vi "ilcbtView.vi"   [LabVIEW 2013, in "ILCBTViews.lvlib"]
uses:
  ILCBTViews.lvlib
  CommandFactory/CommandFactory.lvclass
  UserEvents/UserEvents.lvclass
  UserEvents/UserEvents.lvclass/UserEvents.ctl
  Typedefs/CommandSelector.ctl
  Typedefs/StateSelector.ctl
  Typedefs/ILCBTTypedefs.lvlib
  Controller/Controller.lvclass
  ConfigurationThisComponent/ConfigurationThisComponent.lvclass
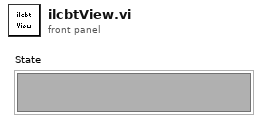
[diagram p1: front panel]
types:
  T1 = enum32{"invalid app kind", "Development System", "Run Time System", "Student Edition", "Embedded LabVIEW", "Evaluation", "Custom"}
  T2 = typedef "ILCBTTypedefs.lvlib/PubDataEvents.ctl" = cluster{"State":refnum<user-event>, "ErrorCode":refnum<user-event>, "OutputData":refnum<user-event>, "LogPath":refnum<user-event>}
  T3 = typedef "ILCBTTypedefs.lvlib/SubDataEvents.ctl" = cluster{"Command":refnum<user-event>}
  T4 = cluster{"Event Registration Refnum":refnum<event-registration>, "Event Registration Refnum":refnum<event-registration>}
  T5 = typedef "ILCBTTypedefs.lvlib/CommandSelector.ctl" = enum16{"ClearError", "Exit", "StandBy", "Start", "Update"}
  T6 = typedef "ILCBTTypedefs.lvlib/StateSelector.ctl" = enum16{"EnabledState", "FaultState", "OffState", "StandbyState"}
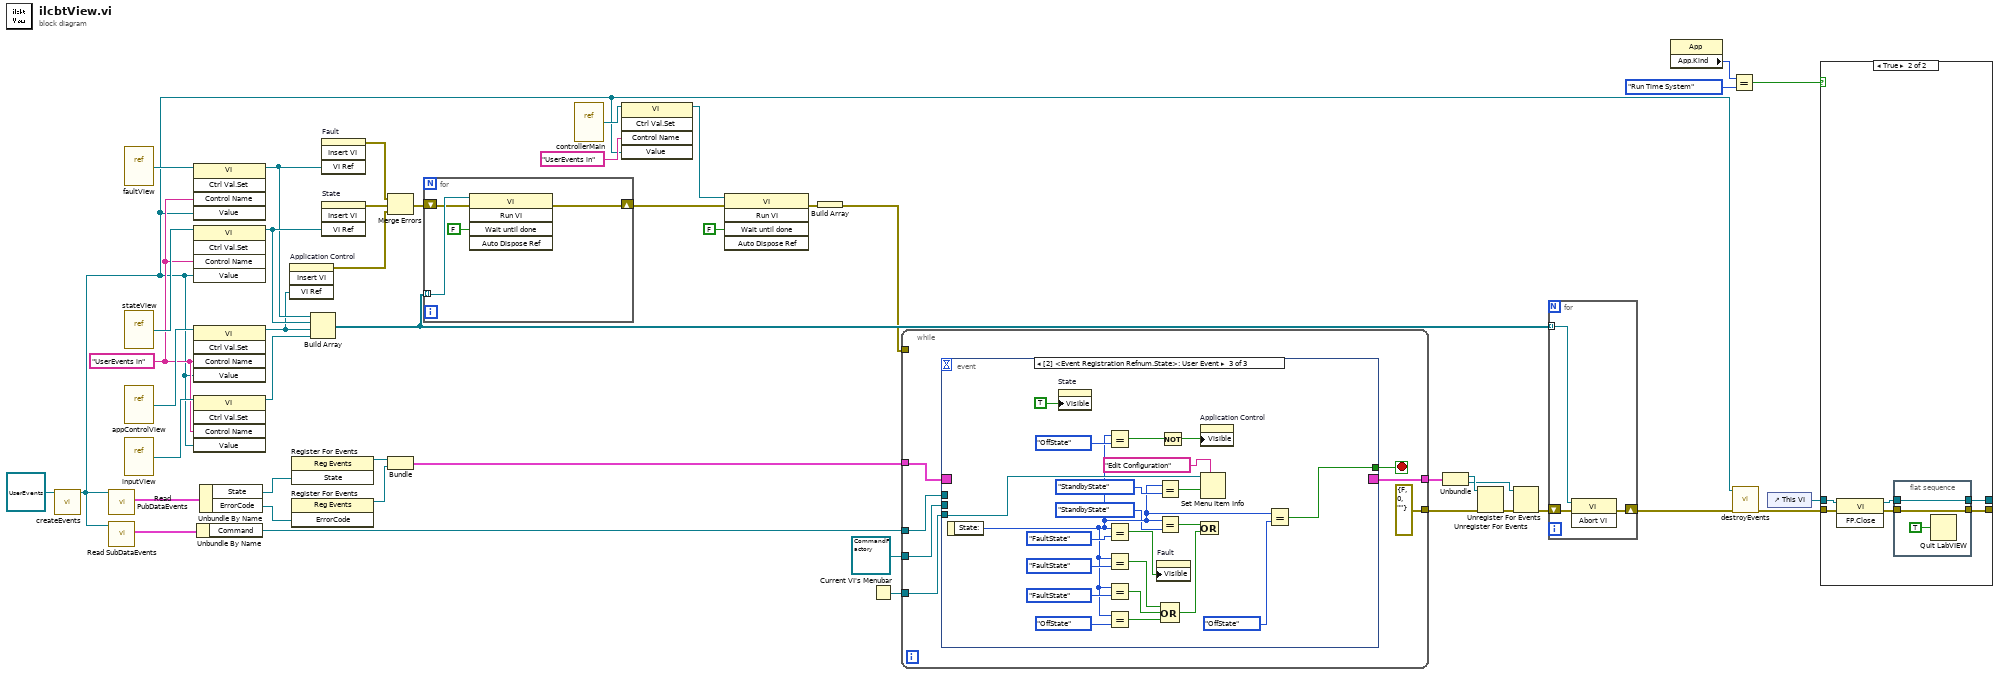
[diagram p0: block diagram]
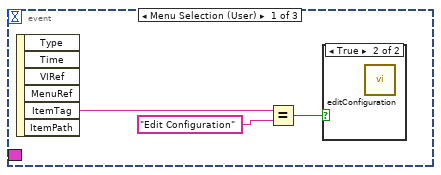
[diagram p3: hidden frame]
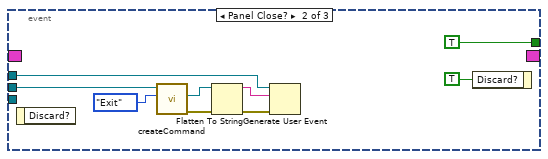
[diagram p5: hidden frame]
diagram:
  w8 = "UserEvents in" ("Control Name")
  n1 = call "createEvents.vi"("UserEvents in"=refnum<class "UserEvents.lvclass"> refnum) -> ("UserEvents out"=w7:refnum<class "UserEvents.lvclass">)  [unwired: 9 in, 1 out]
  n2 = call "Read PubDataEvents.vi"("UserEvents in"=w7) -> ("PubDataEvents"=w38:T2)  [unwired: 9 in, 1 out]
  n3 = call "Read SubDataEvents.vi"("UserEvents in"=w7) -> ("SubDataEvents"=w36:T3)  [unwired: 9 in, 1 out]
  n4 = vi-ref "faultView.vi"() -> (w9:refnum<vi>)
  n5 = vi-ref "stateView.vi"() -> (w12:refnum<vi>)
  n6 = vi-ref "appControlView.vi"() -> (w14:refnum<vi>)
  n7 = vi-ref "inputView.vi"() -> (w26:refnum<vi>)
  n8 = invoke class="VI" method="Ctrl Val.Set"(reference=w9, "Control Name"=w8, "Value"=w7) -> (reference out=w6:refnum<vi>)  [unwired: 2 in, 4 out]
  n9 = invoke class="VI" method="Ctrl Val.Set"(reference=w12, "Control Name"=w8, "Value"=w7) -> (reference out=w11:refnum<vi>)  [unwired: 2 in, 4 out]
  n10 = invoke class="VI" method="Ctrl Val.Set"(reference=w14, "Control Name"=w8, "Value"=w7) -> (reference out=w2:refnum<vi>)  [unwired: 2 in, 4 out]
  n11 = invoke class="VI" method="Ctrl Val.Set"(reference=w26, "Control Name"=w8, "Value"=w7) -> (reference out=w18:refnum<vi>)  [unwired: 2 in, 4 out]
  n12 = Unbundle By Name(w36) -> ("Command"=w35:refnum<user-event>)
  n13 = Unbundle By Name(w38) -> ("State"=w34:refnum<user-event>, "ErrorCode"=w32:refnum<user-event>)
  n14 = invoke on="Application Control" class="SubPnl" method="Insert VI"("VI Ref"=w2) -> (error out=w1:errorcluster)  [unwired: 3 in, 3 out]
  n15 = register-events(w34) -> (reference out=w33:refnum<event-registration>)  [unwired: 2 in, 1 out]
  n16 = register-events(w32) -> (reference out=w31:refnum<event-registration>)  [unwired: 2 in, 1 out]
  n17 = Build Array(w6, w11, w2, w18) -> (w41:refnum<vi>[])
  n18 = invoke on="Fault" class="SubPnl" method="Insert VI"("VI Ref"=w6) -> (error out=w5:errorcluster)  [unwired: 3 in, 3 out]
  n19 = invoke on="State" class="SubPnl" method="Insert VI"("VI Ref"=w11) -> (error out=w10:errorcluster)  [unwired: 3 in, 3 out]
  n20 = Merge Errors(w5, w10, w1) -> (w42:errorcluster)
  n21 = Bundle("Event Registration Refnum"=w33, "Event Registration Refnum"=w31) -> (w24:T4)  [unwired: 1 in]
  n22 = for {
    tunnel: w41 -> [w49] mode=indexing
    shift-right: [w48] -> w13
    shift-left: w42 -> [w47]
    n23 = invoke class="VI" method="Run VI"(reference=w49, error in=w47, "Wait until done"=FALSE ("Wait Until Done")) -> (error out=w48:errorcluster)  [unwired: 2 in, 4 out]
  }
  n24 = vi-ref "controllerMain.vi"() -> (w29:refnum<vi>)
  n25 = invoke class="VI" method="Ctrl Val.Set"(reference=w29, "Control Name"="UserEvents in", "Value"=w7) -> (reference out=w27:refnum<vi>)  [unwired: 2 in, 4 out]
  n26 = invoke class="VI" method="Run VI"(reference=w27, error in=w13, "Wait until done"=FALSE ("Wait Until Done")) -> (error out=w15:errorcluster)  [unwired: 2 in, 4 out]
  n27 = Build Array(w15) -> (w16:errorcluster[])
  n28 = Current VI's Menubar() -> (w39:refnum<k9>)
  n29 = while {
    tunnel: refnum<class "CommandFactory.lvclass"> refnum ("CommandFactory.lvclass") -> [w53]
    tunnel: [errorcluster {"status"=FALSE, "code"=0, "source"=""} ("error out")] -> w25
    tunnel: w39 -> [w51]
    tunnel: w24 -> [w55]
    tunnel: w35 -> [w52]
    tunnel: [w50] -> w23
    tunnel: w16 -> [_]
    stop <- w54 stop-if-true
    n30 = event shown="[2] <Event Registration Refnum.State>: User Event" {
      selector: w55 -> [_ _ _]
      dyn-events: [_ _ _] -> w50
      timeout: _ -> [_ _ _]
      tunnel: [_ TRUE w84] -> w54
      tunnel: w53 -> [_ w63 _]
      tunnel: w52 -> [_ w60 _]
      tunnel: w51 -> [_ _ w86]
      event Menu Selection (User) {
        n31 = event-data() -> ("ItemTag"=w57:string)  [unwired: 1 in, 5 out]
        n32 = Equal?(x=w57, y="Edit Configuration") -> (x = y?=w59:bool)
        n33 = case shown="True" w59 {
          frame False {
          }
          frame True {
            n34 = call "editConfiguration.vi"() -> ()  [unwired: 10 in, 2 out]
          }
        }
      }
      event Panel Close? {
        n35 = event-data() -> ()  [unwired: 1 in, 1 out]
        n36 = call-dynamic "createCommand.vi"("Command"=CommandSelector."Exit", "CommandFactory in"=w63) -> ("error out"=w68:errorcluster, "command"=w67:refnum<class "Command.lvclass">)  [unwired: 7 in, 1 out]
        n37 = Flatten To String(anything=w67, error in (no error)=w68) -> (data string=w61:string, error out=w62:errorcluster)  [unwired: 2 in, 1 out]
        n38 = Generate User Event(user event=w60, event data cluster=w61, error in=w62) -> ()  [unwired: 1 in, 2 out]
        n39 = event-data("Discard?"=TRUE) -> ()  [unwired: 1 in, 1 out]
      }
      event User Event {
        n40 = event-data() -> ("State:"=w80:T6)  [unwired: 1 in]
        n41 = property on="State" class="SubPnl"("Visible"=TRUE) -> ()  [unwired: 2 in, 2 out]
        n42 = Equal?(x=w80, y=StateSelector."OffState") -> (x = y?=w71:bool)
        n43 = Equal?(x=w80, y=StateSelector."FaultState") -> (x = y?=w69:bool)
        n44 = Equal?(x=w80, y=StateSelector."FaultState") -> (x = y?=w78:bool)
        n45 = Equal?(x=w80, y=StateSelector."FaultState") -> (x = y?=w77:bool)
        n46 = Equal?(x=w80, y=StateSelector."OffState") -> (x = y?=w76:bool)
        n47 = property on="Fault" class="SubPnl"("Visible"=w69) -> ()  [unwired: 2 in, 2 out]
        n48 = Equal?(x=w80, y=StateSelector."StandbyState") -> (x = y?=w83:bool)
        n49 = Equal?(x=w80, y=StateSelector."StandbyState") -> (x = y?=w75:bool)
        n50 = Not(x=w71) -> (.not. x?=w72:bool)
        n51 = Compound Arithmetic op=OR(w78, w77, w76) -> (w73:bool)
        n52 = property on="Application Control" class="SubPnl"("Visible"=w72) -> ()  [unwired: 2 in, 2 out]
        n53 = Set Menu Item Info(7:"Edit Configuration" ("item name"), 9:w83, 11:w86) -> ()  [unwired: 4 in, 2 out]
        n54 = Compound Arithmetic op=OR(w75, w73) -> ()  [unwired: 1 out]
        n55 = Equal?(x=w80, y=StateSelector."OffState") -> (x = y?=w84:bool)
      }
    }
  }
  n56 = Unbundle(w23) -> ("Event Registration Refnum"=w22:refnum<event-registration>, "Event Registration Refnum"=w20:refnum<event-registration>)
  n57 = Unregister For Events(event registration refnum=w22, error in=w25) -> (error out=w21:errorcluster)
  n58 = Unregister For Events(event registration refnum=w20, error in=w21) -> (error out=w19:errorcluster)
  n59 = for {
    tunnel: w41 -> [w93] mode=indexing
    shift-right: [w91] -> w17
    shift-left: w19 -> [w92]
    n60 = invoke class="VI" method="Abort VI"(reference=w93, error in=w92) -> (error out=w91:errorcluster)  [unwired: 1 in, 2 out]
  }
  n61 = property class="App"() -> ("App.Kind"=w45:T1)  [unwired: 2 in, 2 out]
  n62 = Equal?(x=w45, y=T1."Run Time System") -> (x = y?=w43:bool)
  n63 = call "destroyEvents.vi"("error in (no error)"=w17, "UserEvents in"=w7) -> ("error out"=w3:errorcluster)  [unwired: 8 in, 1 out]
  n64 = control-ref of="This VI"() -> (w4:refnum<vi>)
  n65 = case shown="True" w43 {
    tunnel: w4 -> [w95 w101]
    tunnel: w3 -> [w94 w100]
    tunnel: [w95 w98] -> _
    tunnel: [w94 w96] -> _
    frame False {
    }
    frame True {
      n66 = invoke class="VI" method="FP.Close"(reference=w101, error in=w100) -> (reference out=w97:refnum<vi>, error out=w99:errorcluster)  [unwired: 1 in, 1 out]
      n67 = flat-sequence {
        tunnel: w99 -> [w102]
        tunnel: [w103] -> w98
        tunnel: w97 -> [w103]
        tunnel: [w102] -> w96
        frame #0 {
          n68 = Quit LabVIEW(quit? (T)=TRUE) -> ()
        }
      }
    }
  }
